vi "SetStageXYTransfer.vi"(8 "error in (no error)":errorcluster, 10 "StageXYTransfer":bool, 11 "Stage_MadCityLab in":refnum<class "Stage_MadCityLab.lvclass">) -> (0 "error out":errorcluster, 3 "Stage_MadCityLab out":refnum<class "Stage_MadCityLab.lvclass">)   [LabVIEW 2020, in "Stage_MadCityLab.lvlib" / "Stage_MadCityLab.lvclass"]
uses:
  Stage_MadCityLab.lvclass
  Stage_MadCityLab.lvclass/Stage_MadCityLab.ctl
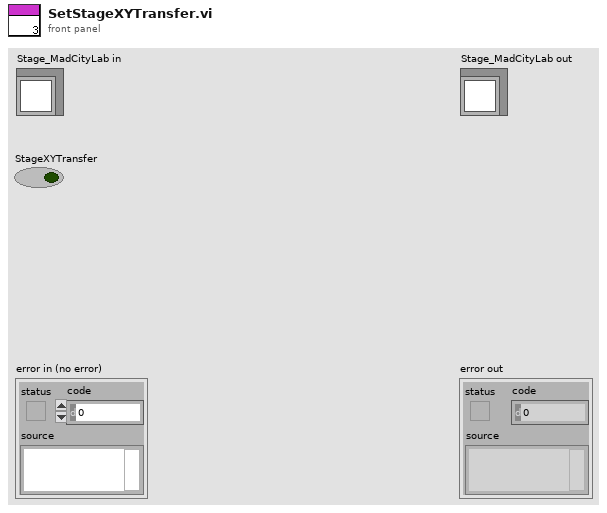
[diagram p1: front panel]
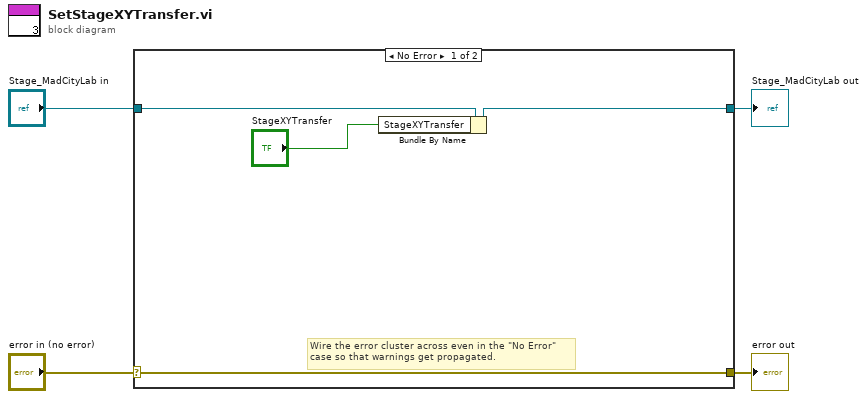
[diagram p0: block diagram]
diagram:
  n1 = case shown="No Error" "error in (no error)" {
    selector: "error in (no error)" -> [w7 w10]
    tunnel: [w7 w10] -> w3
    tunnel: [w6 w9] -> w1
    tunnel: "Stage_MadCityLab in" -> [w8 w9]
    frame No Error {
      # "Wire the error cluster across even in the \"No Error\"\ncase so that warnings get propagated."
      n2 = Bundle By Name(cluster=w8, "StageXYTransfer"="StageXYTransfer") -> (w6:refnum<class "Stage_MadCityLab.lvclass">)
    }
    frame Error {
    }
  }
  "error out" <- w3
  "Stage_MadCityLab out" <- w1
